vi "Get April Tag XY.vi"(7 "Corner":dbl caption="0 = TL, 1 = TR, 2 = BR, 3 = BL", 10 "Detected Tags":T1(array[cluster])) -> (2 "Y":dbl, 3 "X":dbl)   [LabVIEW 2023]
panel:
  in  "Desired tag":dbl
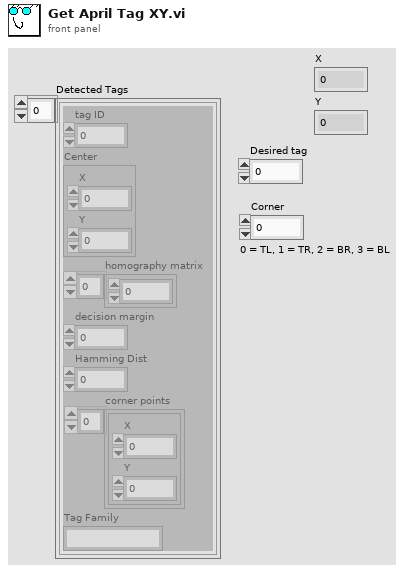
[diagram p1: front panel]
types:
  T1 = cluster{"tag ID":i32, "Center":cluster{"X":dbl, "Y":dbl}, "homography matrix":dbl[], "decision margin":dbl, "Hamming Dist":i32, "corner points":cluster{"X":dbl, "Y":dbl}[], "Tag Family":string}[]
  T2 = cluster{"tag ID":i32, "Center":cluster{"X":dbl, "Y":dbl}, "homography matrix":dbl[], "decision margin":dbl, "Hamming Dist":i32, "corner points":cluster{"X":dbl, "Y":dbl}[], "Tag Family":string}
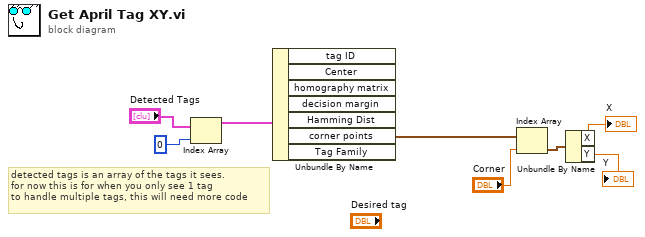
[diagram p0: block diagram]
diagram:
  # "detected tags is an array of the tags it sees. \nfor now this is for when you only see 1 tag\nto handle multiple tags, this will need more code"
  n1 = Index Array(array="Detected Tags", index=0) -> (element=w6:T2)
  n2 = Unbundle By Name(w6) -> ("corner points"=w7:cluster{"X":dbl, "Y":dbl}[])  [unwired: 6 out]
  n3 = Index Array(array=w7, index="Corner") -> (element=w8:cluster{"X":dbl, "Y":dbl})
  n4 = Unbundle By Name(w8) -> ("X"=→"X":dbl, "Y"=→"Y":dbl)
